vi "Single Encode Data.vi"(9 "Tick Constant":dbl, 10 "Rate":dbl, 11 "Distance":dbl) -> (3 "Encoder Values":T1)   [LabVIEW 2016]
uses:
  Common Code/Encoder Values.ctl
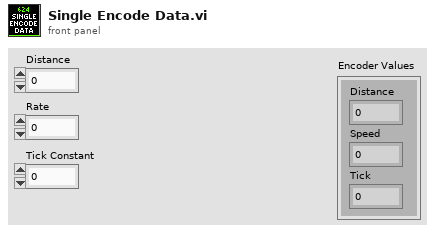
[diagram p1: front panel]
types:
  T1 = typedef "Encoder Values.ctl" = cluster{"Distance":dbl, "Speed":dbl, "Tick":dbl}
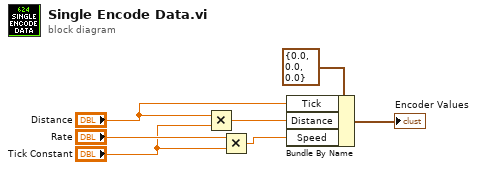
[diagram p0: block diagram]
diagram:
  n1 = Multiply(x="Distance", y="Tick Constant") -> (x*y=w2:dbl)
  n2 = Multiply(x="Rate", y="Tick Constant") -> (x*y=w4:dbl)
  n3 = Bundle By Name(cluster=T1 {"Distance"=0.0, "Speed"=0.0, "Tick"=0.0} ("Encoder Values"), "Tick"="Distance", "Distance"=w2, "Speed"=w4) -> (→"Encoder Values":T1)
